vi "viewDataSocket.vi"() -> ()   [LabVIEW 2009]
panel:
  out "data":variant
  in  "mode":T1(ring)
  out "error out":errorcluster
  in  "URL":string
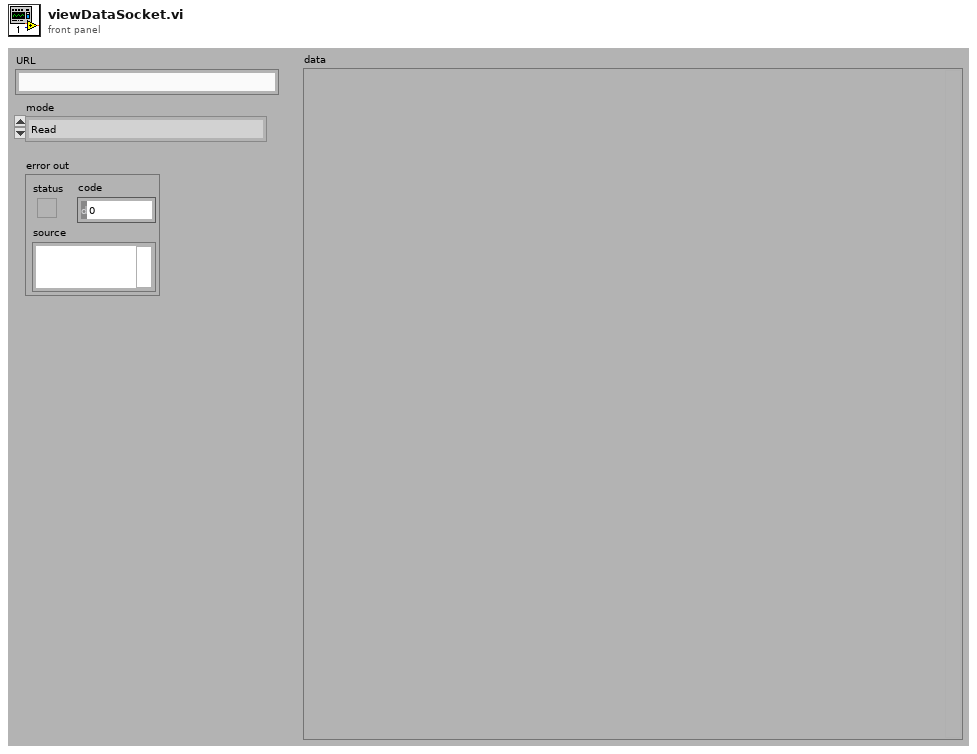
[diagram p1: front panel]
types:
  T1 = enum16{"Read", "Write", "ReadWrite", "BufferedRead", "BufferedReadWrite"}
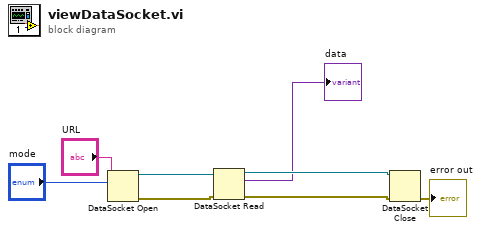
[diagram p0: block diagram]
diagram:
  n1 = DataSocket Open(10:"mode", 11:"URL") -> (0:w5:errorcluster, 3:w6:refnum<k13>)  [unwired: 1 in, 1 out]
  n2 = DataSocket Read(8:w5, 11:w6) -> (0:w3:errorcluster, 2:→"data":variant, 3:w4:refnum<k13>)  [unwired: 7 out]
  n3 = DataSocket Close(8:w3, 11:w4) -> (0:→"error out":errorcluster)  [unwired: 2 out]
